vi "TXT to CSV (BML).vi"() -> ()   [LabVIEW 2016]
uses:
  <vilib>/Utility/file.llb/Read Delimited Spreadsheet (string).vi
panel:
  out "error out":errorcluster
  out "Array":string[][](array[string])
  in  "file path (dialog if empty)":path
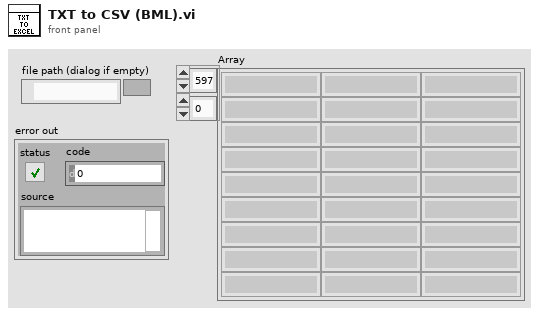
[diagram p1: front panel]
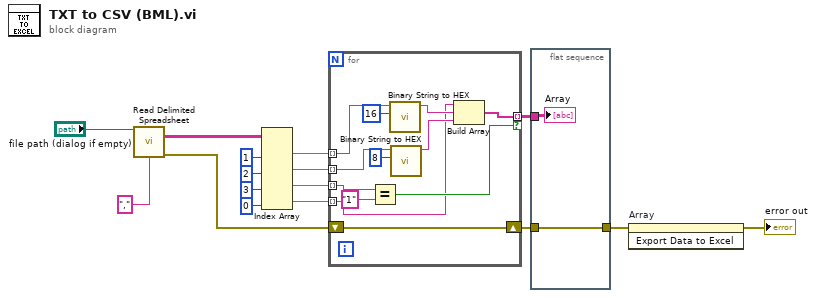
[diagram p0: block diagram]
diagram:
  n1 = call-poly <vilib>:"Read Delimited Spreadsheet.vi"("file path (dialog if empty)"="file path (dialog if empty)", "delimiter (\\t)"="," ("delimiter (\\t)")) -> ("all rows"=w14:string[][], "error out"=w4:errorcluster)  [unwired: 8 in, 4 out]
  n2 = Index Array(array=w14, index (col) #1=1 ("disabled index (col)"), index (col) #2=2 ("index (col)"), index (col) #3=3 ("index (col)"), index (col) #4=0 ("index (col)")) -> (element #1=w10:string[], element #2=w9:string[], element #3=w8:string[], element #4=w5:string[])  [unwired: 4 in]
  n3 = for {
    tunnel: w10 -> [w28] mode=indexing
    tunnel: w9 -> [w26] mode=indexing
    tunnel: w8 -> [w21] mode=indexing
    tunnel: [w22] -> w7 mode=indexing if=w19
    tunnel: w5 -> [w18] mode=indexing
    shift-right: [w17] -> w2
    shift-left: w4 -> [w17]
    n4 = Equal?(x=w21, y="1") -> (x = y?=w19:bool)
    n5 = call "Binary String to HEX.vi"("Bin Length"=16, "Bin String in"=w28) -> ("hex integer string"=w24:string)  [unwired: 9 in]
    n6 = call "Binary String to HEX.vi"("Bin Length"=8, "Bin String in"=w26) -> ("hex integer string"=w23:string)  [unwired: 9 in]
    n7 = Build Array(w18, w24, w23) -> (w22:string[])
  }
  n8 = flat-sequence {
    tunnel: w7 -> [w30]
    tunnel: w2 -> [w29]
    tunnel: [w29] -> w1
    frame #0 {
      "Array" <- w30
    }
  }
  n9 = invoke on="Array" class="Arr (strict)" method="Export Data to Excel"(error in=w1) -> (error out=→"error out":errorcluster)  [unwired: 2 in, 2 out]
